vi "Main_IoT_3.vi"() -> ()   [LabVIEW 2024]
uses:
  <vilib>/LabVIEW Open Source Project/MQTT Control Packets/Control Packets/CONNECT/ConnectFlags -- cluster.ctl
  <vilib>/LabVIEW Open Source Project/MQTT Control Packets/Control Packets/CONNACK/Connect Return Code -- enum.ctl
  CaseControl.ctl
  <vilib>/LabVIEW Open Source Project/MQTT Control Packets/Control Packets/ControlPacket/QualityOfService -- enum.ctl
  <vilib>/LabVIEW Open Source Project/MQTT Client/Client class/Client.lvclass/Client.ctl
  <vilib>/LabVIEW Open Source Project/MQTT Secured TCP Connection/Connection.SecuredTCP/Connection.TCP-TLS.lvclass
  C:/Program Files (x86)/National Instruments/LabVIEW 2024/vi.lib/LabVIEW Open Source Project/Connection/Connection/Connection.lvclass
  <vilib>/LabVIEW Open Source Project/MQTT Client/Client class/Client.lvclass
  C:/Program Files (x86)/National Instruments/LabVIEW 2024/vi.lib/LabVIEW Open Source Project/MQTT Connection/MQTT_Base/Base Class/MQTT_Base.lvclass
  <vilib>/LabVIEW Open Source Project/MQTT Control Packets/Control Packets/PUBLISH/PUBLISH.lvclass
  <vilib>/LabVIEW Open Source Project/MQTT Connection/MQTT_Base/Base Class/MQTT_Base.lvclass
  <vilib>/LabVIEW Open Source Project/MQTT Control Packets/Control Packets/ControlPacket/ControlPacket.lvclass
  <vilib>/LabVIEW Open Source Project/MQTT Control Packets/Control Packets/CONNECT/CONNECT.lvclass
  <vilib>/LabVIEW Open Source Project/MQTT Control Packets/Control Packets/CONNACK/CONNACK.lvclass
panel:
  in  "Server X.509 Certificate":path
  out "Ready for SSL":bool
  out "error out":errorcluster
  out "Return Code":T1=enum."Server Unavailable"
  in  "Payload 2":T2
  in  "Connect Flags":T3={"Reserved"=FALSE, "Clean Session"=TRUE, "Will Flag"=FALSE, "Will QoS 1"=FALSE, "Will QoS 2"=FALSE, "Will Retain"=FALSE, "Password Flag"=FALSE, "User Name Flag"=FALSE}
  in  "Message":string
  out "Published":bool
  in  "Topic Name (empty: Payload name)":string
  in  "Error in":errorcluster
  in  "remote port":u16=80
  in  "address":string="localhost"
  in  "Send Data":bool
  in  "stop":bool
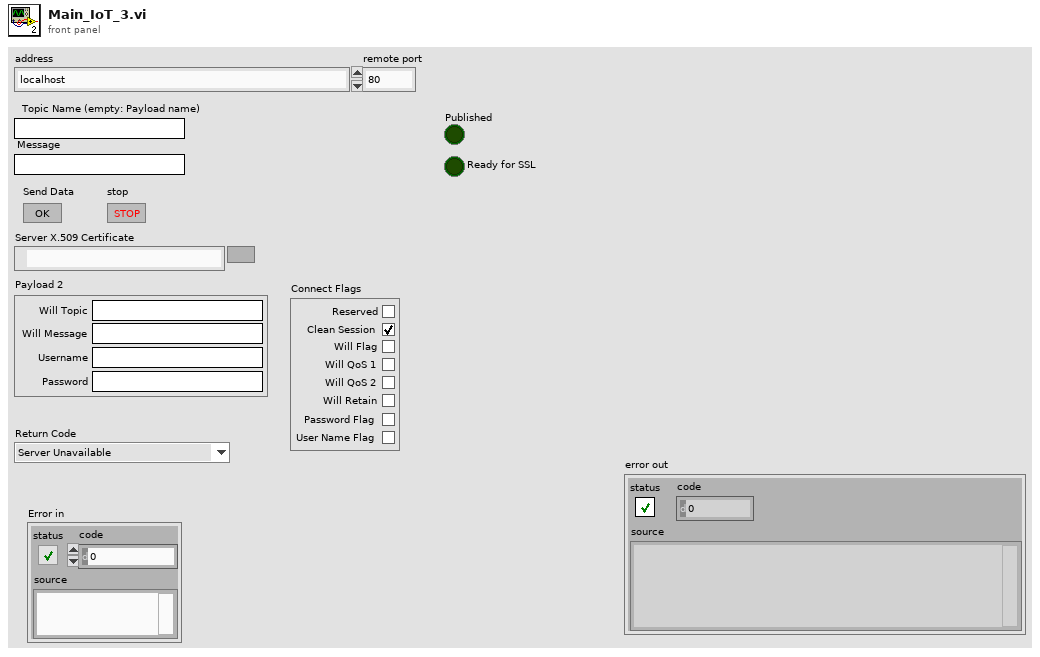
[diagram p1: front panel]
types:
  T1 = typedef "MQTT_Control_Packets.lvlib/CONNACK.lvclass/Connect Return Code -- enum.ctl" = enum16{"Connection accepted", "Unacceptable protocol version", "Identifier Rejected", "Server Unavailable", "Bad Username or Password", "Not Authorized"}
  T2 = cluster{"Will Topic":string, "Will Message":string, "Username":string, "Password":string}
  T3 = typedef "MQTT_Control_Packets.lvlib/CONNECT.lvclass/ConnectFlags -- cluster.ctl" = cluster{"Reserved":bool, "Clean Session":bool, "Will Flag":bool, "Will QoS 1":bool, "Will QoS 2":bool, "Will Retain":bool, "Password Flag":bool, "User Name Flag":bool}
  T4 = typedef "CaseControl.ctl" = enum16{"Init", "Wait", "Publish", "Read", "Exit"}
  T5 = typedef "MQTT_Control_Packets.lvlib/ControlPacket.lvclass/QualityOfService -- enum.ctl" = enum16{"0 (At Most Once)", "1 (At Least Once)", "2 (Exactly Once)"}
  T6 = typedef "MQTT Client.lvlib/Client.lvclass/Public Events -- cluster.ctl" = cluster{"Connection Status":refnum<user-event>, "Connected":refnum<user-event>, "Application Message":refnum<user-event>}
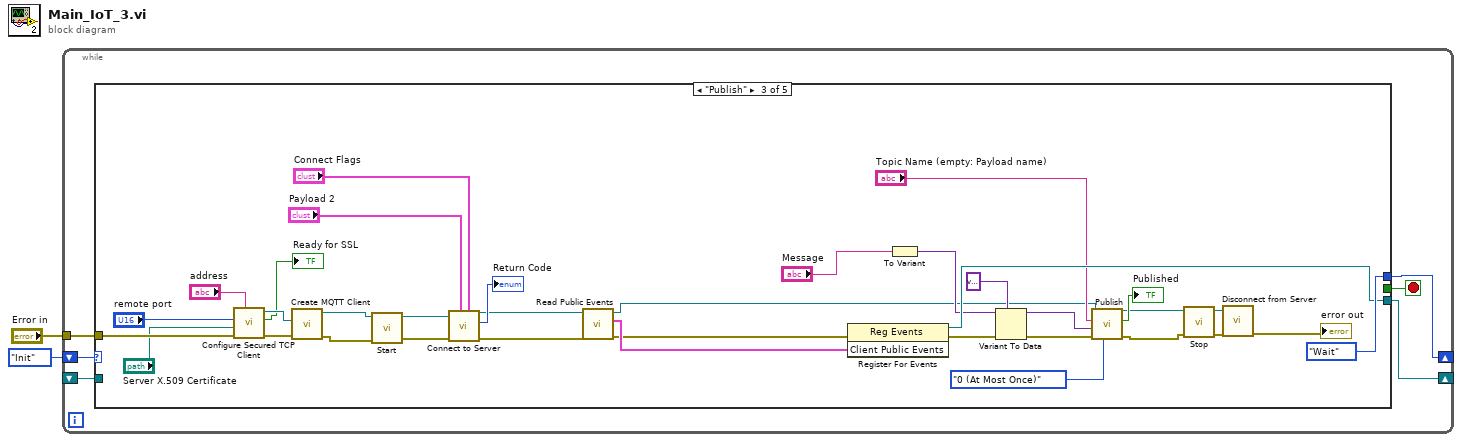
[diagram p0: block diagram]
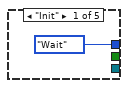
[diagram p2: hidden frame]
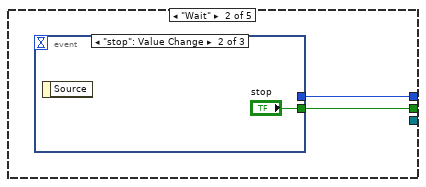
[diagram p3: hidden frame]
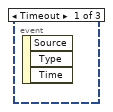
[diagram p4: hidden frame]
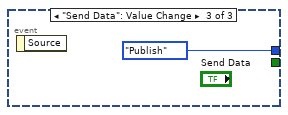
[diagram p5: hidden frame]
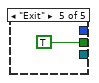
[diagram p7: hidden frame]
diagram:
  n1 = while {
    shift-right: [w7] -> _
    shift-left: CaseControl."Init" ("Case") -> [w8]
    shift-right: [w5] -> _
    shift-left: _ -> [w4]
    tunnel: "Error in" -> [w3]
    stop <- w6 stop-if-true
    n2 = case shown="\"Publish\"" w8 {
      tunnel: [CaseControl."Wait" ("Case") w10 CaseControl."Wait" ("Case") _ _] -> w7
      tunnel: [_ w11 _ _ TRUE ("Boolean")] -> w6
      tunnel: [_ _ w47 _ _] -> w5
      tunnel: w4 -> [_ _ _ _ _]
      tunnel: w3 -> [_ _ w30 _ _]
      frame "Init" {
      }
      frame "Wait" {
        n3 = event shown="[1] \"stop\": Value Change" {
          selector: _ -> [_ _ _]
          dyn-events: _ -> [_ _ _]
          timeout: _ -> [_ _ _]
          tunnel: [_ "stop" _] -> w11
          tunnel: [_ _ CaseControl."Publish" ("Case")] -> w10
          event Timeout {
            n4 = event-data() -> ()  [unwired: 1 in, 3 out]
          }
          event "stop": Value Change {
            n5 = event-data() -> ()  [unwired: 1 in, 1 out]
          }
          event "Send Data": Value Change {
            n6 = event-data() -> ()  [unwired: 1 in, 1 out]
          }
        }
      }
      frame "Publish" {
        n7 = call <vilib>:"Configure Secured TCP Client.vi"("Hostname"="address", "error in (no error)"=w30, "Server X.509 Certificate"="Server X.509 Certificate", "remote port (443)"="remote port") -> ("error out"=w33:errorcluster, "Ready for SSL"=→"Ready for SSL":bool, "Secured TCP Connection"=w34:refnum<class "Connection.TCP-TLS.lvclass">)  [unwired: 5 in]
        n8 = call <vilib>:"Create MQTT Client.vi"("error in (no error)"=w33, "Connection Configuration"=w34) -> ("error out"=w22:errorcluster, "Client out"=w23:refnum<class "Client.lvclass">)  [unwired: 8 in]
        n9 = call <vilib>:"Start.vi"("error in (no error)"=w22, "MQTT_Base in"=w23) -> ("error out"=w24:errorcluster, "MQTT_Base out"=w25:refnum<class "Client.lvclass">)  [unwired: 7 in, 1 out]
        n10 = call <vilib>:"Connect to Server.vi"("Connect Flags"="Connect Flags", "Payload"="Payload 2", "error in (no error)"=w24, "Client in"=w25) -> ("error out"=w21:errorcluster, "Return Code"=→"Return Code":T1, "Client out"=w20:refnum<class "Client.lvclass">)  [unwired: 4 in, 1 out]
        n11 = call <vilib>:"Read Public Events.vi"("error in (no error)"=w21, "Client in"=w20) -> ("error out"=w35:errorcluster, "Client Public Events"=w37:T6, "Client out"=w36:refnum<class "Client.lvclass">)  [unwired: 7 in]
        n12 = register-events(error in=w35, w37) -> (reference out=w47:refnum<event-registration>, error out=w38:errorcluster)  [unwired: 1 in]
        n13 = To Variant(anything="Message") -> (Variant=w41:variant)
        n14 = Variant To Data(error in=w38, type=variant ("Payload"), Variant=w41) -> (data=w39:variant, error out=w40:errorcluster)
        n15 = call <vilib>:"Publish.vi"("QoS"=QualityOfService_--_enum."0 (At Most Once)", "error in (no error)"=w40, "Payload"=w39, "Topic Name (empty: Payload name)"="Topic Name (empty: Payload name)", "Client in"=w36) -> ("error out"=w17:errorcluster, "Published"=→"Published":bool, "Client out"=w16:refnum<class "Client.lvclass">)  [unwired: 4 in]
        n16 = call <vilib>:"Stop.vi"("error in (no error)"=w17, "MQTT_Base in"=w16) -> ("error out"=w18:errorcluster, "MQTT_Base out"=w14:refnum<class "Client.lvclass">)  [unwired: 7 in, 1 out]
        n17 = call <vilib>:"Disconnect from Server.vi"("error in (no error)"=w18, "Client in"=w14) -> ("error out"=→"error out":errorcluster)  [unwired: 7 in, 2 out]
      }
      frame "Read" {
      }
      frame "Exit" {
      }
    }
  }
